vi "SCA-RT.vi"() -> ()   [LabVIEW 2016]
uses:
  controls/state control sample changer.ctl
  <vilib>/Platform/TimedLoop/XDataNode/timing_clust.ctl
  <vilib>/Platform/TimedLoop/XDataNode/nitl_modes.ctl
  <vilib>/Platform/TimedLoop/XDataNode/wakeup.ctl
  <vilib>/Analysis/baseanly.llb/Mean (DBL).vi
  <vilib>/Instr/_visa.llb/VISA Configure Serial Port (Instr).vi
  <vilib>/Motion/Express/_s/nimc.fb.read.readExecutionData.axis.vi
  <vilib>/Platform/TimedLoop/XDataNode/loadnilvce.vi
  <vilib>/Motion/Express/_s/nimc.fb.straightLineMove.startStraightLineMove.axis.modeAbsolute.0.vi
  <vilib>/Motion/Express/_s/nimc.fb.straightLineMove.startStraightLineMove.axis.modeRelative.0.vi
  <vilib>/Motion/BlockNode/FB.NIMotion.xnode
  <vilib>/Platform/TimedLoop/XDataNode/XDataNode.xnode
  <vilib>/Platform/TimedLoop/XDataNode/XDNodeRunTimeDep.lvlib
  <resource>/objmgr/nimcca.rc
  <vilib>/Analysis/NI_AALBase.lvlib
panel:
  out "Sample Rod DOWN":bool
  out "Sample Rod UP":bool
  out "SC GV CLOSED":bool
  out "SC GV OPEN":bool
  out "Retract Rod IN":bool
  out "Retract Rod OUT":bool
  out "Insert Rod IN":bool
  out "Insert Rod OUT":bool
  out "sample rod UP sensor":bool
  out "sample rod DOWN sensor":bool
  out "SC GV OPEN sensor":bool
  out "SC GV CLOSED sensor":bool
  out "insert rod IN sensor":bool
  out "insert rod OUT sensor":bool
  out "retract rod IN sensor":bool
  out "retract rod OUT sensor":bool
  out "Bellows IG 2":dbl
  out "Bellows CG 2":dbl
  out "Bellows CG 1":dbl
  out "Source CG 2":dbl
  out "Source CG 1":dbl
  out "Source IG1":dbl
  out "Bellows IG 1":dbl
  out "Source IG2":dbl
  out "CV 4":string
  out "CV 3":string
  out "ig 4":string
  out "ig 3":string
  out "CV 2":string
  out "CV 1":string
  out "ig 2":string
  out "cathode change":bool
  out "extractor current read":dbl
  out "extractor voltage read":dbl
  out "extractor set":dbl
  out "cathode voltage read":dbl
  out "cathode current":dbl
  out "cathode set":dbl
  in  "execute":bool
  out "Move (motor steps)":dbl
  out "Destination (encoder)":dbl
  in  "Window radius":u32=2
  out "In Range?":bool
  out "Lower Limit":u32
  out "Upper Limit":u32
  out "encoder position":u16
  out "change sample start end":bool
  out "start sample change":bool
  in  "clear error 3":bool
  in  "clear error 2":bool
  out "encoder set value":dbl
  out "done 2":bool
  out "set rod down 2":bool
  out "set cold cathode on 2":bool
  out "rotate wheel":bool
  out "set cold cathode on":bool
  out "set cold cathode off":bool
  out "set  vent source":bool
  out "set pump out system":bool
  out "set push out rod in":bool
  out "set push out rod out":bool
  out "set sc open":bool
  out "set sc close":bool
  out "set insert in":bool
  out "set insert out":bool
  out "set rod down":bool
  out "set rod up":bool
  out "Strings []":string[](array[string])
  out "wheel position readback":dbl
  out "position":dbl
  in  "clear error":bool
  out "action":string
  out "Axis Index":i32
  in  "end sample test":bool
  out "ig 1":string
  out "error out 8":errorcluster
  out "ig2":string
  out "error out 5":errorcluster
  out "convec":string
  out "Rod Up error out":errorcluster
  out "Retract Out 1 error out":errorcluster
  out "Retract In 1 error out":errorcluster
  out "indextest":dbl
  out "sc control":T1
  out "done":bool
  out "error out":errorcluster
  out "state control 2":T1
  in  "state control":T1="wait"
  in  "New Sample":dbl=1.0
  # "State Machine Sensors"
  # "Sensor Monitor Loop"
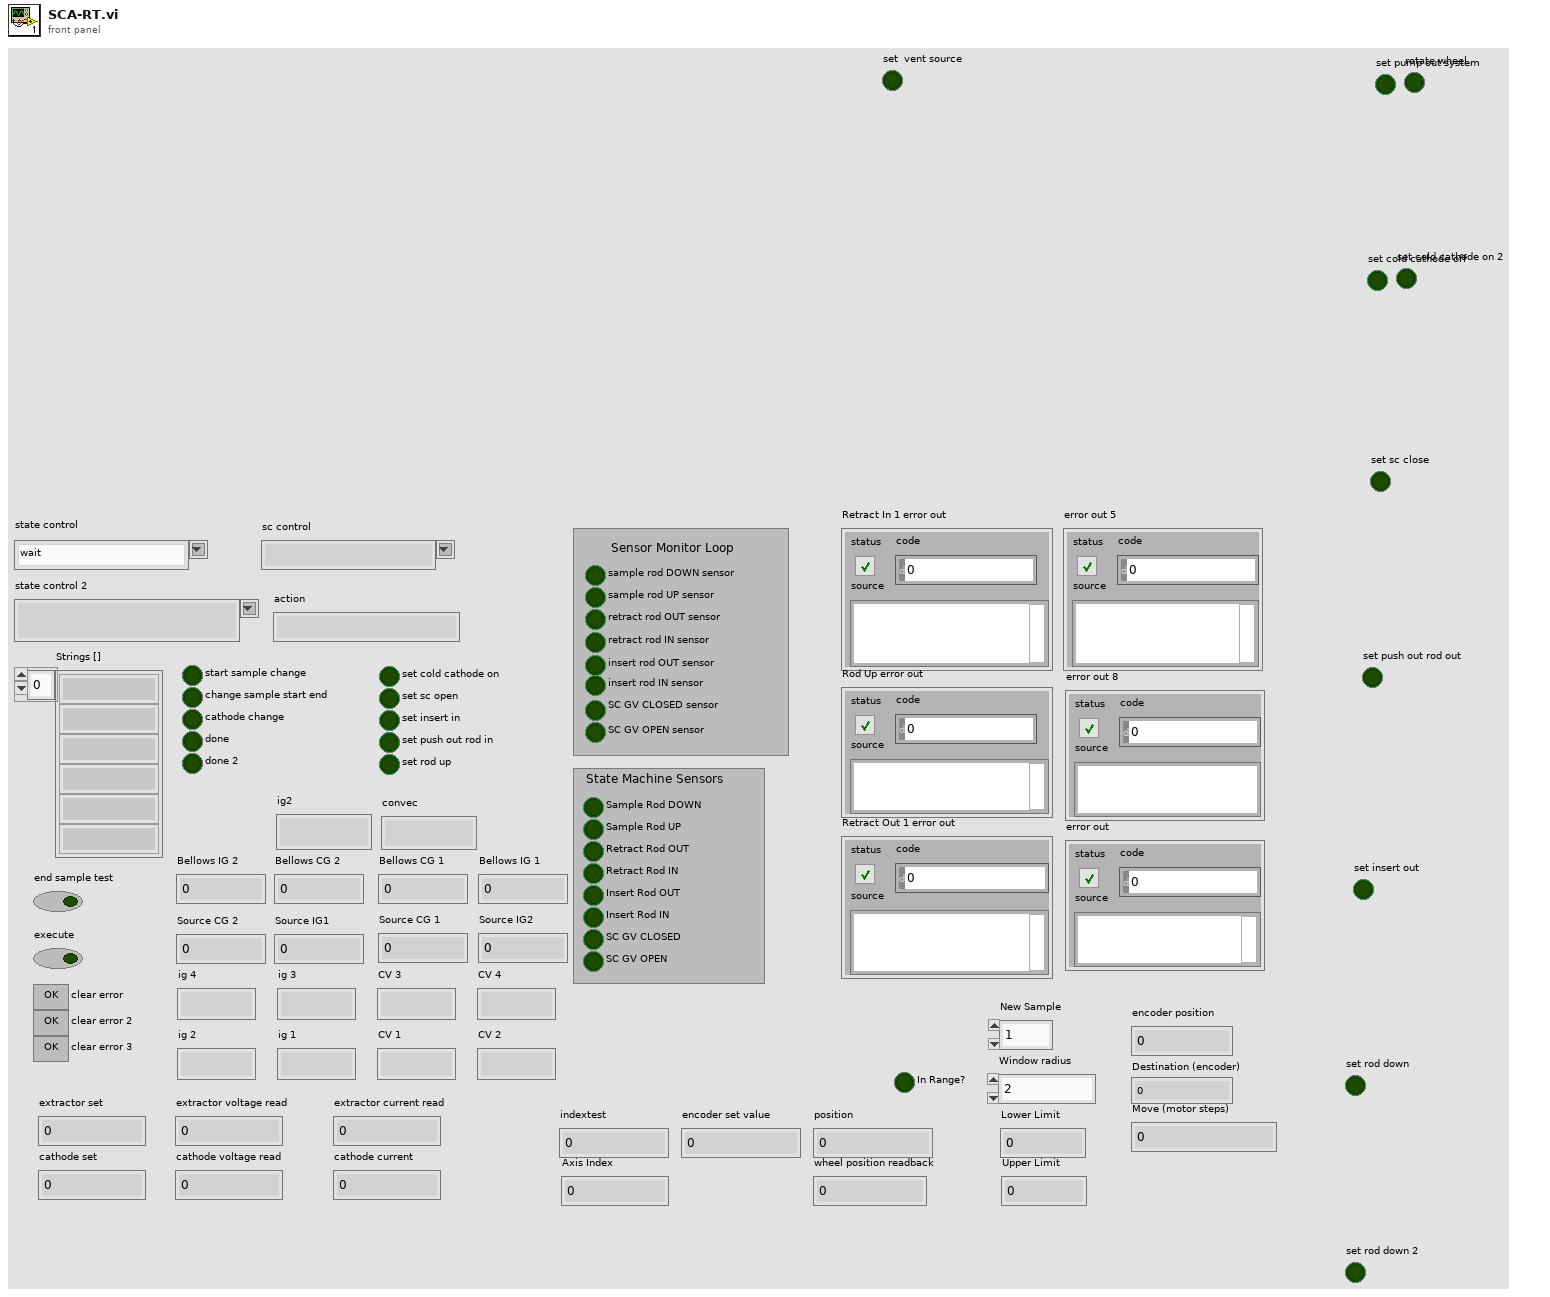
[diagram p1: front panel]
types:
  T1 = typedef "state control sample changer.ctl" = string
  T2 = typedef "XDNodeRunTimeDep.lvlib/timing_clust.ctl" = cluster{"Expected End [f-1]":u64, "Actual End [f-1]":u64, "Finished Late? [f-1]":bool, "Expected End [i-1]":u64, "Actual End [i-1]":u64, "Finished Late? [i-1]":bool, "Expected Start [i]":u64, "Actual Start [i]":u64, "Expected Start [f]":u64, "Actual Start [f]":u64, "Source Name":string, "Structure Name":string, "Period":i64, "Deadline":i64, "Offset":i64, "Start":i64, "Priority":i32, "Timeout":i32, "Mode":T3, "Wakeup Reason":T4, "Error":errorcluster, "Source Type":string, "Secondary Source Type":string, "Global End Time":u64, "Global Start Time":u64, "Frame Duration":u64, "Iteration Duration":u64, "Assigned CPU":i32, "I/O Scan Engine Mode":u32}
  T3 = typedef "XDNodeRunTimeDep.lvlib/nitl_modes.ctl" = enum32{"No Change", "Process missed periods, maintain original phase", "Discard missed periods, maintain original phase", "Process missed periods, ignore original phase", "Discard missed periods, ignore original phase"}
  T4 = typedef "XDNodeRunTimeDep.lvlib/wakeup.ctl" = enum32{"Normal", "Aborted", "Asynchronous wakeup", "Timing source error", "Timed loop error", "Timeout"}
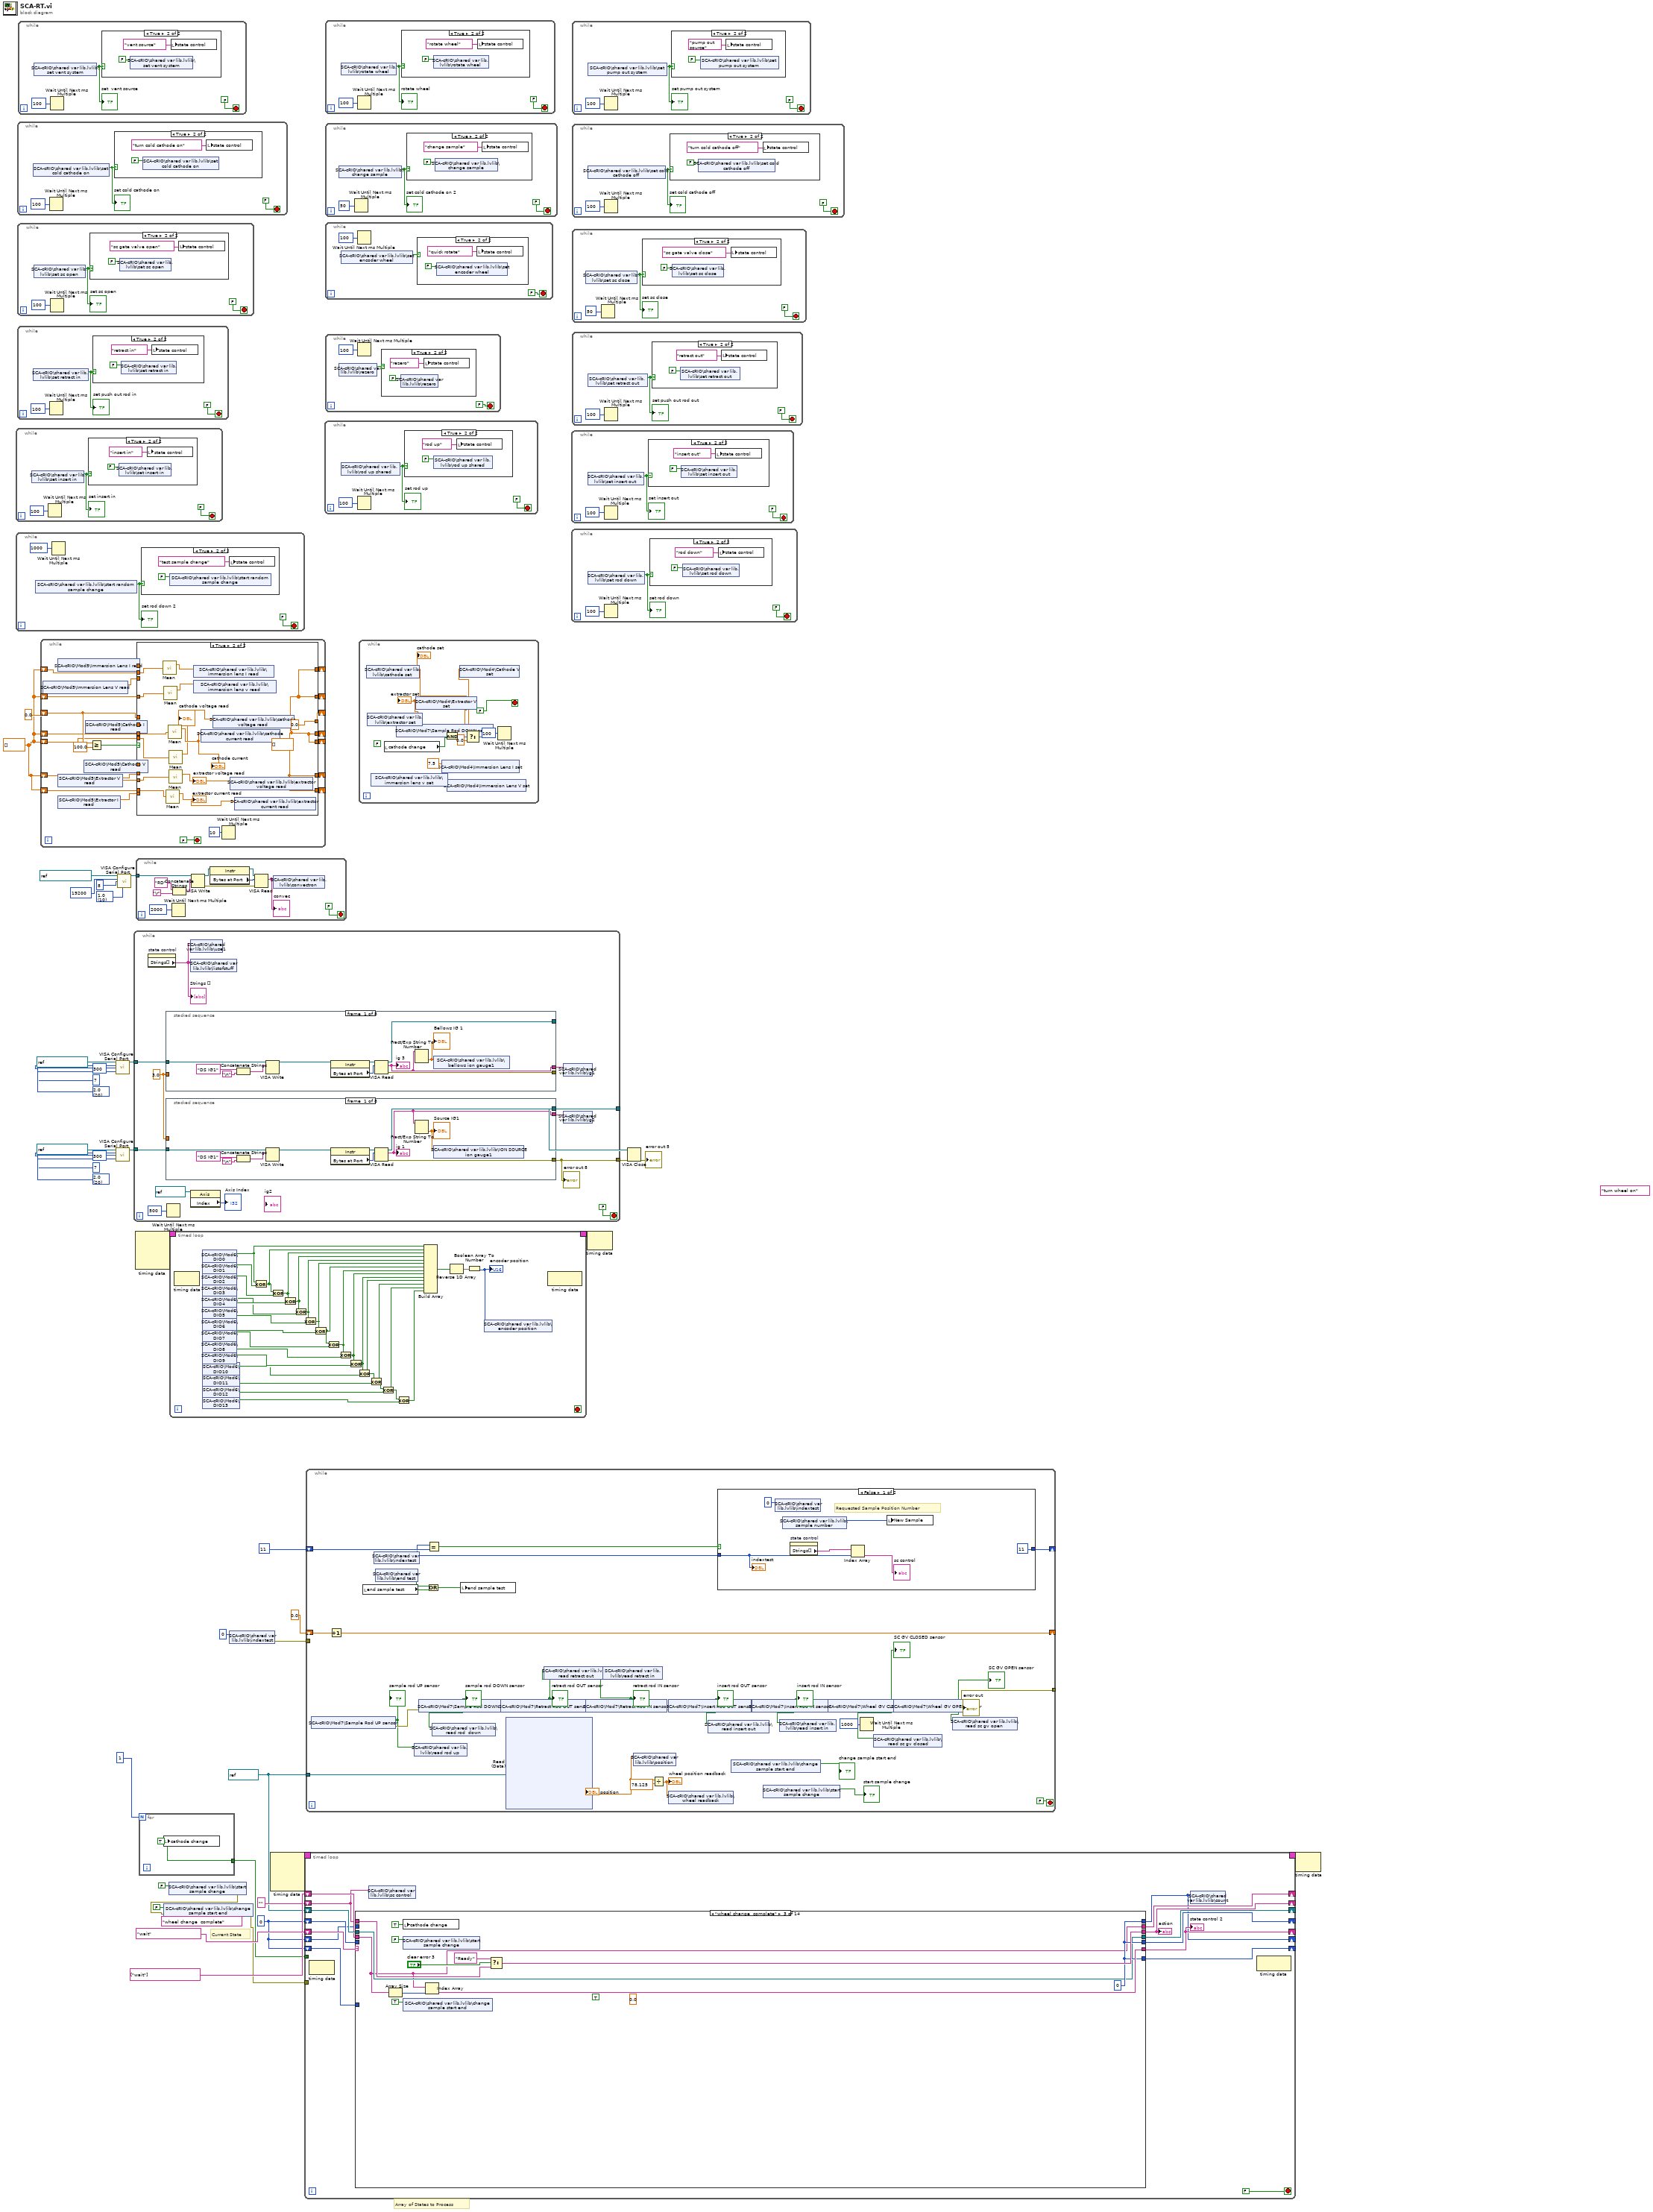
[diagram p0: block diagram]
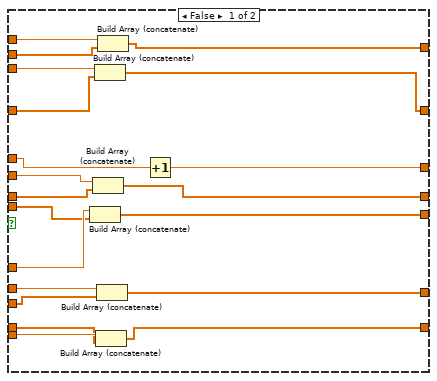
[diagram p2: hidden frame]
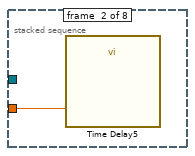
[diagram p20: hidden frame]
diagram:
  w1 = dbl[] []
  (unwired) T1 "wheel change  complete" ("state control")
  (unwired) T1 "turn wheel on" ("state control")
  w28 = u16 20 items=["1.0"=10, "1.5"=15, "2.0"=20] ("stop bits (10: 1 bit)")
  w32 = u16 10 items=["1.0"=10, "1.5"=15, "2.0"=20] ("stop bits (10: 1 bit)")
  w19 = u16 20 items=["1.0"=10, "1.5"=15, "2.0"=20] ("stop bits (10: 1 bit)")
  w13 = 0
  w12 = refnum<k21> "Axis 1" ("resource")
  # "Current State"
  # "Array of States to Process"
  n1 = while {
    stop <- FALSE stop-if-true
    n2 = shared-variable "SCA-cRIO\\shared var lib.lvlib\\set insert in"() -> (w41:bool)  [unwired: 1 in, 1 out]
    "set insert in" <- w41
    n3 = Wait Until Next ms Multiple(millisecond multiple=u32 100) -> ()  [unwired: 1 out]
    n4 = case shown="True" w41 {
      frame False {
      }
      frame True {
        n5 = shared-variable "SCA-cRIO\\shared var lib.lvlib\\set insert in"(FALSE ("rod up shared")) -> ()  [unwired: 1 in, 1 out]
        n6 = local write "state control"(T1 "insert in" ("state control")) -> ()
      }
    }
  }
  n7 = while {
    stop <- FALSE stop-if-true
    n8 = shared-variable "SCA-cRIO\\shared var lib.lvlib\\start random sample change"() -> (w46:bool)  [unwired: 1 in, 1 out]
    "set rod down 2" <- w46
    n9 = Wait Until Next ms Multiple(millisecond multiple=u32 1000) -> ()  [unwired: 1 out]
    n10 = case shown="True" w46 {
      frame False {
      }
      frame True {
        n11 = shared-variable "SCA-cRIO\\shared var lib.lvlib\\start random sample change"(FALSE ("rod up shared")) -> ()  [unwired: 1 in, 1 out]
        n12 = local write "state control"(T1 "test sample change" ("state control")) -> ()
      }
    }
  }
  n13 = while {
    stop <- FALSE stop-if-true
    n14 = shared-variable "SCA-cRIO\\shared var lib.lvlib\\set cold cathode on"() -> (w51:bool)  [unwired: 1 in, 1 out]
    "set cold cathode on" <- w51
    n15 = Wait Until Next ms Multiple(millisecond multiple=u32 100) -> ()  [unwired: 1 out]
    n16 = case shown="True" w51 {
      frame False {
      }
      frame True {
        n17 = shared-variable "SCA-cRIO\\shared var lib.lvlib\\set cold cathode on"(FALSE ("rod up shared")) -> ()  [unwired: 1 in, 1 out]
        n18 = local write "state control"(T1 "turn cold cathode on" ("state control")) -> ()
      }
    }
  }
  n19 = while {
    stop <- FALSE stop-if-true
    n20 = shared-variable "SCA-cRIO\\shared var lib.lvlib\\set retract in"() -> (w56:bool)  [unwired: 1 in, 1 out]
    "set push out rod in" <- w56
    n21 = Wait Until Next ms Multiple(millisecond multiple=u32 100) -> ()  [unwired: 1 out]
    n22 = case shown="True" w56 {
      frame False {
      }
      frame True {
        n23 = shared-variable "SCA-cRIO\\shared var lib.lvlib\\set retract in"(FALSE ("rod up shared")) -> ()  [unwired: 1 in, 1 out]
        n24 = local write "state control"(T1 "retract in" ("state control")) -> ()
      }
    }
  }
  n25 = while {
    stop <- FALSE stop-if-true
    n26 = shared-variable "SCA-cRIO\\shared var lib.lvlib\\set sc open"() -> (w61:bool)  [unwired: 1 in, 1 out]
    "set sc open" <- w61
    n27 = Wait Until Next ms Multiple(millisecond multiple=u32 100) -> ()  [unwired: 1 out]
    n28 = case shown="True" w61 {
      frame False {
      }
      frame True {
        n29 = shared-variable "SCA-cRIO\\shared var lib.lvlib\\set sc open"(FALSE ("rod up shared")) -> ()  [unwired: 1 in, 1 out]
        n30 = local write "state control"(T1 "sc gate valve open" ("state control")) -> ()
      }
    }
  }
  n31 = while {
    stop <- FALSE stop-if-true
    n32 = shared-variable "SCA-cRIO\\shared var lib.lvlib\\set vent system"() -> (w66:bool)  [unwired: 1 in, 1 out]
    "set  vent source" <- w66
    n33 = Wait Until Next ms Multiple(millisecond multiple=u32 100) -> ()  [unwired: 1 out]
    n34 = case shown="True" w66 {
      frame False {
      }
      frame True {
        n35 = shared-variable "SCA-cRIO\\shared var lib.lvlib\\set vent system"(FALSE ("rod up shared")) -> ()  [unwired: 1 in, 1 out]
        n36 = local write "state control"(T1 "vent source" ("state control")) -> ()
      }
    }
  }
  n37 = while {
    shift-right: [w86] -> _
    shift-left: 0.0 ("AI1") -> [w89]
    shift-right: [w84] -> _
    shift-left: w1 -> [w83]
    shift-right: [w85] -> _
    shift-left: w1 -> [w82]
    shift-right: [w80] -> _
    shift-left: w1 -> [w79]
    shift-right: [w77] -> _
    shift-left: w1 -> [w76]
    shift-right: [w71] -> _
    shift-left: w1 -> [w74]
    shift-right: [w70] -> _
    shift-left: w1 -> [w75]
    stop <- FALSE stop-if-true
    n38 = shared-variable "SCA-cRIO\\Mod5\\Immersion Lens V read"() -> (w72:dbl)  [unwired: 1 in, 1 out]
    n39 = shared-variable "SCA-cRIO\\Mod5\\Extractor V read"() -> (w81:dbl)  [unwired: 1 in, 1 out]
    n40 = shared-variable "SCA-cRIO\\Mod5\\Extractor I read"() -> (w78:dbl)  [unwired: 1 in, 1 out]
    n41 = shared-variable "SCA-cRIO\\Mod5\\Immersion Lens I read"() -> (w73:dbl)  [unwired: 1 in, 1 out]
    n42 = shared-variable "SCA-cRIO\\Mod5\\Cathode V read"() -> (w91:dbl)  [unwired: 1 in, 1 out]
    n43 = shared-variable "SCA-cRIO\\Mod5\\Cathode I read"() -> (w90:dbl)  [unwired: 1 in, 1 out]
    n44 = Greater Or Equal?(x=w89, y=100.0) -> (x >= y?=w87:bool)
    n45 = case shown="True" w87 {
      tunnel: w91 -> [w109 _]
      tunnel: w90 -> [w110 _]
      tunnel: w89 -> [w113 _]
      tunnel: [w112 0.0 ("AI1")] -> w86
      tunnel: [w111 w116] -> w85
      tunnel: [w108 w116] -> w84
      tunnel: w83 -> [w107 w125]
      tunnel: w82 -> [w106 w126]
      tunnel: w81 -> [w105 _]
      tunnel: [w104 w116] -> w80
      tunnel: w79 -> [w103 w124]
      tunnel: w78 -> [w102 _]
      tunnel: [w101 w116] -> w77
      tunnel: w76 -> [w100 w123]
      tunnel: w75 -> [w99 w115]
      tunnel: w74 -> [w98 w114]
      tunnel: w73 -> [w97 _]
      tunnel: w72 -> [w96 _]
      tunnel: [w95 w116] -> w71
      tunnel: [w94 w116] -> w70
      frame False {
        n46 = Build Array (concatenate)(w109, w107) -> (w108:dbl[])
        n47 = Build Array (concatenate)(w110, w106) -> (w111:dbl[])
        n48 = Build Array (concatenate)(w96, w99) -> (w94:dbl[])
        n49 = Build Array (concatenate)(w102, w100) -> (w101:dbl[])
        n50 = Build Array (concatenate)(w105, w103) -> (w104:dbl[])
        n51 = Build Array (concatenate)(w97, w98) -> (w95:dbl[])
        n52 = Increment(x=w113) -> (x+1=w112:dbl)
      }
      frame True {
        w116 = dbl[] []
        n53 = call-poly <vilib>:"Mean.vi"("X"=w114) -> ("mean"=w117:dbl)  [unwired: 1 out]
        n54 = call-poly <vilib>:"Mean.vi"("X"=w115) -> ("mean"=w118:dbl)  [unwired: 1 out]
        n55 = call-poly <vilib>:"Mean.vi"("X"=w123) -> ("mean"=w119:dbl)  [unwired: 1 out]
        "extractor current read" <- w119
        n56 = call-poly <vilib>:"Mean.vi"("X"=w126) -> ("mean"=w122:dbl)  [unwired: 1 out]
        "cathode current" <- w122
        n57 = call-poly <vilib>:"Mean.vi"("X"=w124) -> ("mean"=w120:dbl)  [unwired: 1 out]
        "extractor voltage read" <- w120
        n58 = call-poly <vilib>:"Mean.vi"("X"=w125) -> ("mean"=w121:dbl)  [unwired: 1 out]
        "cathode voltage read" <- w121
        n59 = shared-variable "SCA-cRIO\\shared var lib.lvlib\\immersion lens I read"(w117) -> ()  [unwired: 1 in, 1 out]
        n60 = shared-variable "SCA-cRIO\\shared var lib.lvlib\\immersion lens v read"(w118) -> ()  [unwired: 1 in, 1 out]
        n61 = shared-variable "SCA-cRIO\\shared var lib.lvlib\\cathode current read"(w122) -> ()  [unwired: 1 in, 1 out]
        n62 = shared-variable "SCA-cRIO\\shared var lib.lvlib\\cathode voltage read"(w121) -> ()  [unwired: 1 in, 1 out]
        n63 = shared-variable "SCA-cRIO\\shared var lib.lvlib\\extractor voltage read"(w120) -> ()  [unwired: 1 in, 1 out]
        n64 = shared-variable "SCA-cRIO\\shared var lib.lvlib\\extractor current read"(w119) -> ()  [unwired: 1 in, 1 out]
      }
    }
    n65 = Wait Until Next ms Multiple(millisecond multiple=u32 10) -> ()  [unwired: 1 out]
  }
  n66 = call-poly "VISA Configure Serial Port"("VISA resource name"=refnum<visa-resource-name> "ASRL8::INSTR", "baud rate (9600)"=u32 300, "data bits (8)"=u16 7, "stop bits (10: 1 bit)"=w28) -> ("VISA resource name out"=w29:refnum<visa-resource-name>)  [unwired: 10 in, 1 out]
  n67 = call-poly "VISA Configure Serial Port"("VISA resource name"=refnum<visa-resource-name> "ASRL6::INSTR", "baud rate (9600)"=u32 300, "data bits (8)"=u16 7, "stop bits (10: 1 bit)"=w19) -> ("VISA resource name out"=w20:refnum<visa-resource-name>)  [unwired: 10 in, 1 out]
  n68 = call-poly "VISA Configure Serial Port"("VISA resource name"=refnum<visa-resource-name> "ASRL7::INSTR", "baud rate (9600)"=u32 19200, "data bits (8)"=u16 8, "stop bits (10: 1 bit)"=w32) -> ("VISA resource name out"=w15:refnum<visa-resource-name>)  [unwired: 10 in, 1 out]
  n69 = while {
    tunnel: w20 -> [w138]
    tunnel: [w137] -> w21
    tunnel: [w136] -> w22
    tunnel: w29 -> [w130]
    stop <- FALSE ("stop 4") stop-if-true
    w129 = 3.0 ("Delay Time (s)")
    n70 = property on="state control" class="CmbBox (strict)"() -> ("Strings[]"=w132:string[])  [unwired: 2 in, 2 out]
    "Strings []" <- w132
    n71 = stacked-sequence {
      tunnel: w130 -> [w150 _ w160 _ w170 _ w180 _]
      tunnel: [w147 _ _ _ _ _ _ _] -> _
      tunnel: [w146 _ _ _ _ _ _ _] -> _
      tunnel: [w141 _ _ _ _ _ _ _] -> w128
      tunnel: w129 -> [_ w151 _ w161 _ w171 _ w181]
      frame #0 {
        n72 = Concatenate Strings("DS IG1" ("write buffer"), "\n") -> (w142:string)
        n73 = VISA Write(VISA resource name=w150, write buffer=w142) -> (VISA resource name out=w149:refnum<visa-resource-name>)  [unwired: 1 in, 2 out]
        n74 = property class="Instr"(reference=w149) -> (reference out=w148:refnum<visa-resource-name>, "Bytes at Port"=w144:u32)  [unwired: 1 in, 1 out]
        n75 = VISA Read(VISA resource name=w148, byte count=w144) -> (VISA resource name out=w147:refnum<visa-resource-name>, read buffer=w141:string, error out=w146:errorcluster)  [unwired: 1 in, 1 out]
        "ig 3" <- w141
        n76 = Fract/Exp String To Number(string=w141) -> (number=w140:dbl)  [unwired: 3 in, 1 out]
        "Bellows IG 1" <- w140
        n77 = shared-variable "SCA-cRIO\\shared var lib.lvlib\\bellows ion gauge1"(w140) -> ()  [unwired: 1 in, 1 out]
      }
      frame #1 {
        n78 = call "Time Delay5"("Delay Time (s)"=w151) -> ()  [unwired: 10 in, 1 out]
      }
      frame #2 {
        n79 = Concatenate Strings("DS IG2" ("write buffer"), "\n") -> (w154:string)
        n80 = VISA Write(VISA resource name=w160, write buffer=w154) -> (VISA resource name out=w159:refnum<visa-resource-name>)  [unwired: 1 in, 2 out]
        n81 = property class="Instr"(reference=w159) -> (reference out=w158:refnum<visa-resource-name>, "Bytes at Port"=w156:u32)  [unwired: 1 in, 1 out]
        n82 = VISA Read(VISA resource name=w158, byte count=w156) -> (read buffer=w153:string)  [unwired: 1 in, 3 out]
        "ig 4" <- w153
        n83 = Fract/Exp String To Number(string=w153) -> (number=w152:dbl)  [unwired: 3 in, 1 out]
        "Bellows IG 2" <- w152
        n84 = shared-variable "SCA-cRIO\\shared var lib.lvlib\\bellows ion gauge2"(w152) -> ()  [unwired: 1 in, 1 out]
      }
      frame #3 {
        n85 = call "Time Delay6"("Delay Time (s)"=w161) -> ()  [unwired: 10 in, 1 out]
      }
      frame #4 {
        n86 = Concatenate Strings("DS CG1" ("write buffer"), "\n") -> (w164:string)
        n87 = VISA Write(VISA resource name=w170, write buffer=w164) -> (VISA resource name out=w169:refnum<visa-resource-name>)  [unwired: 1 in, 2 out]
        n88 = property class="Instr"(reference=w169) -> (reference out=w168:refnum<visa-resource-name>, "Bytes at Port"=w166:u32)  [unwired: 1 in, 1 out]
        n89 = VISA Read(VISA resource name=w168, byte count=w166) -> (read buffer=w163:string)  [unwired: 1 in, 3 out]
        "CV 3" <- w163
        n90 = Fract/Exp String To Number(string=w163) -> (number=w162:dbl)  [unwired: 3 in, 1 out]
        "Bellows CG 1" <- w162
        n91 = shared-variable "SCA-cRIO\\shared var lib.lvlib\\Bellows covectron1"(w162) -> ()  [unwired: 1 in, 1 out]
      }
      frame #5 {
        n92 = call "Time Delay7"("Delay Time (s)"=w171) -> ()  [unwired: 10 in, 1 out]
      }
      frame #6 {
        n93 = Concatenate Strings("DS CG2" ("write buffer"), "\n") -> (w174:string)
        n94 = VISA Write(VISA resource name=w180, write buffer=w174) -> (VISA resource name out=w179:refnum<visa-resource-name>)  [unwired: 1 in, 2 out]
        n95 = property class="Instr"(reference=w179) -> (reference out=w178:refnum<visa-resource-name>, "Bytes at Port"=w176:u32)  [unwired: 1 in, 1 out]
        n96 = VISA Read(VISA resource name=w178, byte count=w176) -> (read buffer=w173:string)  [unwired: 1 in, 3 out]
        "CV 4" <- w173
        n97 = Fract/Exp String To Number(string=w173) -> (number=w172:dbl)  [unwired: 3 in, 1 out]
        "Bellows CG 2" <- w172
        n98 = shared-variable "SCA-cRIO\\shared var lib.lvlib\\Bellows covectron2"(w172) -> ()  [unwired: 1 in, 1 out]
      }
      frame #7 {
        n99 = call "Time Delay8"("Delay Time (s)"=w181) -> ()  [unwired: 10 in, 1 out]
      }
    }
    n100 = stacked-sequence {
      tunnel: w138 -> [w192 _ w202 _ w212 _ w222 _]
      tunnel: [w189 _ _ _ _ _ _ _] -> w137
      tunnel: [w188 _ _ _ _ _ _ _] -> w136
      tunnel: [w183 _ _ _ _ _ _ _] -> w131
      tunnel: w129 -> [_ w193 _ w203 _ w213 _ w223]
      frame #0 {
        n101 = Concatenate Strings("DS IG1" ("write buffer"), "\n") -> (w184:string)
        n102 = VISA Write(VISA resource name=w192, write buffer=w184) -> (VISA resource name out=w191:refnum<visa-resource-name>)  [unwired: 1 in, 2 out]
        n103 = property class="Instr"(reference=w191) -> (reference out=w190:refnum<visa-resource-name>, "Bytes at Port"=w186:u32)  [unwired: 1 in, 1 out]
        n104 = VISA Read(VISA resource name=w190, byte count=w186) -> (VISA resource name out=w189:refnum<visa-resource-name>, read buffer=w183:string, error out=w188:errorcluster)  [unwired: 1 in, 1 out]
        "ig 1" <- w183
        n105 = Fract/Exp String To Number(string=w183) -> (number=w182:dbl)  [unwired: 3 in, 1 out]
        "Source IG1" <- w182
        n106 = shared-variable "SCA-cRIO\\shared var lib.lvlib\\ION SOURCE ion gauge1"(w182) -> ()  [unwired: 1 in, 1 out]
      }
      frame #1 {
        n107 = call "Time Delay3"("Delay Time (s)"=w193) -> ()  [unwired: 10 in, 1 out]
      }
      frame #2 {
        n108 = Concatenate Strings("DS IG2" ("write buffer"), "\n") -> (w196:string)
        n109 = VISA Write(VISA resource name=w202, write buffer=w196) -> (VISA resource name out=w201:refnum<visa-resource-name>)  [unwired: 1 in, 2 out]
        n110 = property class="Instr"(reference=w201) -> (reference out=w200:refnum<visa-resource-name>, "Bytes at Port"=w198:u32)  [unwired: 1 in, 1 out]
        n111 = VISA Read(VISA resource name=w200, byte count=w198) -> (read buffer=w195:string)  [unwired: 1 in, 3 out]
        "ig 2" <- w195
        n112 = Fract/Exp String To Number(string=w195) -> (number=w194:dbl)  [unwired: 3 in, 1 out]
        "Source IG2" <- w194
        n113 = shared-variable "SCA-cRIO\\shared var lib.lvlib\\ION SOURCE ion gauge2"(w194) -> ()  [unwired: 1 in, 1 out]
      }
      frame #3 {
        n114 = call "Time Delay"("Delay Time (s)"=w203) -> ()  [unwired: 10 in, 1 out]
      }
      frame #4 {
        n115 = Concatenate Strings("DS CG1" ("write buffer"), "\n") -> (w206:string)
        n116 = VISA Write(VISA resource name=w212, write buffer=w206) -> (VISA resource name out=w211:refnum<visa-resource-name>)  [unwired: 1 in, 2 out]
        n117 = property class="Instr"(reference=w211) -> (reference out=w210:refnum<visa-resource-name>, "Bytes at Port"=w208:u32)  [unwired: 1 in, 1 out]
        n118 = VISA Read(VISA resource name=w210, byte count=w208) -> (read buffer=w205:string)  [unwired: 1 in, 3 out]
        "CV 1" <- w205
        n119 = Fract/Exp String To Number(string=w205) -> (number=w204:dbl)  [unwired: 3 in, 1 out]
        "Source CG 1" <- w204
        n120 = shared-variable "SCA-cRIO\\shared var lib.lvlib\\ION SOURCE covectron1"(w204) -> ()  [unwired: 1 in, 1 out]
      }
      frame #5 {
        n121 = call "Time Delay2"("Delay Time (s)"=w213) -> ()  [unwired: 10 in, 1 out]
      }
      frame #6 {
        n122 = Concatenate Strings("DS CG2" ("write buffer"), "\n") -> (w216:string)
        n123 = VISA Write(VISA resource name=w222, write buffer=w216) -> (VISA resource name out=w221:refnum<visa-resource-name>)  [unwired: 1 in, 2 out]
        n124 = property class="Instr"(reference=w221) -> (reference out=w220:refnum<visa-resource-name>, "Bytes at Port"=w218:u32)  [unwired: 1 in, 1 out]
        n125 = VISA Read(VISA resource name=w220, byte count=w218) -> (read buffer=w215:string)  [unwired: 1 in, 3 out]
        "CV 2" <- w215
        n126 = Fract/Exp String To Number(string=w215) -> (number=w214:dbl)  [unwired: 3 in, 1 out]
        "Source CG 2" <- w214
        n127 = shared-variable "SCA-cRIO\\shared var lib.lvlib\\ION SOURCE covectron2"(w214) -> ()  [unwired: 1 in, 1 out]
      }
      frame #7 {
        n128 = call "Time Delay4"("Delay Time (s)"=w223) -> ()  [unwired: 10 in, 1 out]
      }
    }
    "error out 8" <- w136
    n129 = Wait Until Next ms Multiple(millisecond multiple=u32 500) -> ()  [unwired: 1 out]
    n130 = shared-variable "SCA-cRIO\\shared var lib.lvlib\\use1"(w132) -> ()  [unwired: 1 in, 1 out]
    n131 = shared-variable "SCA-cRIO\\shared var lib.lvlib\\listofstuff"(w132) -> ()  [unwired: 1 in, 1 out]
    n132 = property class="Axis"(reference=refnum<k21> "Axis 1" ("resource")) -> ("Index"=→"Axis Index":i32)  [unwired: 1 in, 2 out]
    n133 = shared-variable "SCA-cRIO\\shared var lib.lvlib\\ig1"(w128) -> ()  [unwired: 1 in, 1 out]
    n134 = shared-variable "SCA-cRIO\\shared var lib.lvlib\\ig2"(w131) -> ()  [unwired: 1 in, 1 out]
  }
  n135 = node-c288() -> (w6:T2)  [unwired: 4 in]
  n136 = while {
    tunnel: w15 -> [w226]
    stop <- FALSE ("stop 3") stop-if-true
    n137 = Wait Until Next ms Multiple(millisecond multiple=u32 2000) -> ()  [unwired: 1 out]
    n138 = Concatenate Strings("RD" ("write buffer 2"), "\r") -> (w234:string)
    n139 = VISA Write(VISA resource name=w226, write buffer=w234) -> (VISA resource name out=w228:refnum<visa-resource-name>, error out=w227:errorcluster)  [unwired: 1 in, 1 out]
    n140 = property class="Instr"(reference=w228) -> (reference out=w229:refnum<visa-resource-name>, "Bytes at Port"=w230:u32)  [unwired: 1 in, 1 out]
    n141 = VISA Read(VISA resource name=w229, byte count=w230, error in (no error)=w227) -> (read buffer=w224:string)  [unwired: 3 out]
    "convec" <- w224
    n142 = shared-variable "SCA-cRIO\\shared var lib.lvlib\\convectron"(w224) -> ()  [unwired: 1 in, 1 out]
  }
  n143 = for {
    N: 1 -> [_]
    tunnel: [w235] -> w2
    w235 = TRUE ("cathode change")
    n144 = local write "cathode change"(w235) -> ()
  }
  n145 = shared-variable "SCA-cRIO\\shared var lib.lvlib\\start sample change"(FALSE ("start sample change")) -> (error out=w8:errorcluster)  [unwired: 1 in]
  n146 = shared-variable "SCA-cRIO\\shared var lib.lvlib\\change sample start end"(FALSE ("change sample start end"), error in=w8) -> (error out=w7:errorcluster)
  n147 = timed-loop {
    timing: w6 -> [_]
    timing-out: [_] -> w5
    stop <- _ stop-if-true
    n148 = node-c288() -> ()  [unwired: 1 in, 1 out]
    n149 = shared-variable "SCA-cRIO\\Mod6\\DIO0"() -> (w252:bool)  [unwired: 1 in, 1 out]
    n150 = shared-variable "SCA-cRIO\\Mod6\\DIO1"() -> (w251:bool)  [unwired: 1 in, 1 out]
    n151 = shared-variable "SCA-cRIO\\Mod6\\DIO2"() -> (w250:bool)  [unwired: 1 in, 1 out]
    n152 = shared-variable "SCA-cRIO\\Mod6\\DIO3"() -> (w249:bool)  [unwired: 1 in, 1 out]
    n153 = shared-variable "SCA-cRIO\\Mod6\\DIO4"() -> (w248:bool)  [unwired: 1 in, 1 out]
    n154 = shared-variable "SCA-cRIO\\Mod6\\DIO5"() -> (w247:bool)  [unwired: 1 in, 1 out]
    n155 = shared-variable "SCA-cRIO\\Mod6\\DIO6"() -> (w246:bool)  [unwired: 1 in, 1 out]
    n156 = shared-variable "SCA-cRIO\\Mod6\\DIO7"() -> (w245:bool)  [unwired: 1 in, 1 out]
    n157 = shared-variable "SCA-cRIO\\Mod6\\DIO8"() -> (w244:bool)  [unwired: 1 in, 1 out]
    n158 = shared-variable "SCA-cRIO\\Mod6\\DIO9"() -> (w243:bool)  [unwired: 1 in, 1 out]
    n159 = shared-variable "SCA-cRIO\\Mod6\\DIO10"() -> (w242:bool)  [unwired: 1 in, 1 out]
    n160 = shared-variable "SCA-cRIO\\Mod6\\DIO11"() -> (w241:bool)  [unwired: 1 in, 1 out]
    n161 = shared-variable "SCA-cRIO\\Mod6\\DIO12"() -> (w240:bool)  [unwired: 1 in, 1 out]
    n162 = shared-variable "SCA-cRIO\\Mod6\\DIO13"() -> (w239:bool)  [unwired: 1 in, 1 out]
    n163 = Exclusive Or(1:w251, 2:w252) -> (0:w253:bool)
    n164 = Exclusive Or(1:w250, 2:w253) -> (0:w254:bool)
    n165 = Exclusive Or(1:w249, 2:w254) -> (0:w255:bool)
    n166 = Exclusive Or(1:w248, 2:w255) -> (0:w256:bool)
    n167 = Exclusive Or(1:w247, 2:w256) -> (0:w257:bool)
    n168 = Exclusive Or(1:w246, 2:w257) -> (0:w258:bool)
    n169 = Exclusive Or(1:w245, 2:w258) -> (0:w259:bool)
    n170 = Exclusive Or(1:w244, 2:w259) -> (0:w260:bool)
    n171 = Exclusive Or(1:w243, 2:w260) -> (0:w261:bool)
    n172 = Exclusive Or(1:w242, 2:w261) -> (0:w262:bool)
    n173 = Exclusive Or(1:w241, 2:w262) -> (0:w263:bool)
    n174 = Exclusive Or(1:w240, 2:w263) -> (0:w264:bool)
    n175 = Exclusive Or(1:w239, 2:w264) -> (0:w265:bool)
    n176 = Build Array(w252, w253, w254, w255, w256, w257, w258, w259, w260, w261, w262, w263, w264, w265) -> (w237:bool[])
    n177 = Reverse 1D Array(array=w237) -> (reversed array=w236:bool[])
    n178 = Boolean Array To Number(Boolean array=w236) -> (number=w238:u32)
    "encoder position" <- w238
    n179 = shared-variable "SCA-cRIO\\shared var lib.lvlib\\encoder position"(w238) -> ()  [unwired: 1 in, 1 out]
    n180 = node-c288() -> ()  [unwired: 1 in, 1 out]
  }
  n181 = shared-variable "SCA-cRIO\\shared var lib.lvlib\\indextest"(i16 0 ("indextest")) -> (error out=w33:errorcluster)  [unwired: 1 in]
  n182 = node-c288() -> (w39:T2)  [unwired: 4 in]
  n183 = timed-loop {
    timing: w39 -> [_]
    timing-out: [_] -> w38
    shift-right: [w280] -> _
    shift-left: w12 -> [w281]
    shift-right: [w278] -> _
    shift-left: T1 "wait" ("state control") -> [w279]
    shift-right: [w274] -> _
    shift-left: T1[] ["wait"] -> [w277]
    shift-right: [w275] -> _
    shift-left: w13 -> [w276]
    shift-right: [w273] -> _
    shift-left: "" -> [w270]
    shift-right: [w271] -> _
    shift-left: w13 -> [w272]
    shift-right: [w268] -> _
    shift-left: w13 -> [w269]
    tunnel: w7 -> [_]
    tunnel: w2 -> [_]
    stop <- FALSE ("stop 2") stop-if-true
    n184 = node-c288() -> ()  [unwired: 1 in, 1 out]
    n185 = case shown="\"wheel change  complete\"" w279 {
      selector: w279 -> [_ _ _ w378 w420 w449 w487 w523 _ _ w613 w677 w743 w767]
      tunnel: w281 -> [w293 w353 w365 w400 w438 w476 w512 w542 w558 w609 w640 w681 w728 w788]
      tunnel: [w293 w353 w365 w400 w438 w476 w512 w542 w557 w609 w639 w681 w728 w787] -> w280
      tunnel: [w283 w359 w371 w381 w422 w453 w492 w529 w556 w599 w629 w679 w744 w768] -> w278
      tunnel: w277 -> [w292 w351 w362 w379 w421 w448 w488 w522 w555 w611 w614 w676 w704 w771]
      tunnel: w276 -> [_ _ _ w388 w432 w463 w500 _ _ w605 w636 w693 w726 w783]
      tunnel: [w286 w354 w366 w387 w428 w460 w499 w532 w553 w604 w637 w694 w726 w784] -> w275
      tunnel: [w284 w351 w362 w382 w412 w456 w491 w530 w555 w611 w630 w690 w746 w770] -> w274
      tunnel: w270 -> [w289 w357 w369 _ _ _ _ _ _ _ _ _ _ _]
      tunnel: [w288 w356 w368 w377 w424 w455 w490 w538 "wheel off" ("y") "sample changer test" ("y") w628 w689 w742 w766] -> w273
      tunnel: w272 -> [_ _ _ w383 w419 w452 w495 w536 _ _ w631 w691 _ w772]
      tunnel: [w286 w354 w366 w376 w415 w451 w494 w527 w553 0 w622 w684 0 ("t") w760] -> w271
      tunnel: w269 -> [_ _ _ w375 w414 w450 w489 w526 w552 w592 w627 w688 w741 w765]
      tunnel: [w286 w354 w366 w375 w414 w450 w489 w526 w552 w591 w627 w688 w741 w765] -> w268
      frame "wait", Default {
        w286 = 0
        n186 = Select(t="Ready", s="clear error", f=w289) -> (s? t:f=w288:string)
        n187 = case shown="\"rod up\"" "state control" {
          tunnel: w292 -> [_ _ _ _ _ _ _ _ _ _ _ _ _ _ _ _ _ _]
          tunnel: [w294 w297 w300 w303 w306 w309 w312 w315 w318 w321 w325 w328 w331 w334 w337 w339 w342 w347] -> w284
          tunnel: "state control" -> [_ _ _ _ _ _ _ _ _ _ _ _ _ _ _ _ _ _]
          tunnel: [w295 w298 w301 w304 w307 w310 w313 w316 w319 w322 w324 w327 w330 w333 w336 w340 w343 w345] -> _
          frame "sc gate valve close" {
            w294 = T1[] ["sc gate valve close"]
            n188 = Index Array(array=w294, index=0) -> (element=w295:T1)
          }
          frame "sc gate valve open" {
            w297 = T1[] ["sc gate valve open"]
            n189 = Index Array(array=w297, index=0) -> (element=w298:T1)
          }
          frame "rod up" {
            w300 = T1[] ["rod up"]
            n190 = Index Array(array=w300, index=0) -> (element=w301:T1)
          }
          frame "rod down" {
            w303 = T1[] ["rod down"]
            n191 = Index Array(array=w303, index=0) -> (element=w304:T1)
          }
          frame "retract in" {
            w306 = T1[] ["retract in"]
            n192 = Index Array(array=w306, index=0) -> (element=w307:T1)
          }
          frame "retract out" {
            w309 = T1[] ["retract out"]
            n193 = Index Array(array=w309, index=0) -> (element=w310:T1)
          }
          frame "insert in" {
            w312 = T1[] ["insert in"]
            n194 = Index Array(array=w312, index=0) -> (element=w313:T1)
          }
          frame "insert out" {
            w315 = T1[] ["insert out"]
            n195 = Index Array(array=w315, index=0) -> (element=w316:T1)
          }
          frame "turn cold cathode on" {
            w318 = T1[] ["turn cold cathode on"]
            n196 = Index Array(array=w318, index=0) -> (element=w319:T1)
          }
          frame "turn cold cathode off" {
            w321 = T1[] ["turn cold cathode off"]
            n197 = Index Array(array=w321, index=0) -> (element=w322:T1)
          }
          frame "rotate wheel" {
            w325 = T1[] ["check position"]
            n198 = Index Array(array=w325, index=0) -> (element=w324:T1)
          }
          frame "change sample" {
            w328 = T1[] ["wheel change start", "rod up", "retract in", "retract out", "check position", "insert in", "insert out", "rod down", "wheel change  complete"]
            n199 = Index Array(array=w328, index=0) -> (element=w327:T1)
          }
          frame "test sample change" {
            w331 = T1[] ["rod up", "retract in", "retract out", "check position", "insert in", "insert out", "rod down", "test sample change"]
            n200 = Index Array(array=w331, index=0) -> (element=w330:T1)
          }
          frame "vent source" {
            w334 = T1[] ["turn cold cathode off", "rod up", "retract in", "retract out", "insert out", "sc gate valve close"]
            n201 = Index Array(array=w334, index=0) -> (element=w333:T1)
          }
          frame "pump out source" {
            w337 = T1[] ["sc gate valve open", "rod up", "check position", "insert in", "insert out", "rod down"]
            n202 = Index Array(array=w337, index=0) -> (element=w336:T1)
          }
          frame "wait", Default {
            w339 = T1[] ["wait"]
            n203 = Index Array(array=w339, index=0) -> (element=w340:T1)
          }
          frame "quick rotate" {
            w342 = T1[] ["quick rotate"]
            n204 = Index Array(array=w342, index=0) -> (element=w343:T1)
          }
          frame "rezero" {
            w347 = T1[] ["rezero"]
            n205 = Index Array(array=w347, index=0) -> (element=w345:T1)
          }
        }
        n206 = Index Array(array=w284, index=0) -> (element=w283:T1)
      }
      frame "wheel change start" {
        (unwired) 0.0 ("position")
        w354 = 0
        n207 = shared-variable "SCA-cRIO\\shared var lib.lvlib\\start sample change"(TRUE ("start sample change")) -> ()  [unwired: 1 in, 1 out]
        n208 = shared-variable "SCA-cRIO\\shared var lib.lvlib\\change sample start end"(FALSE ("change sample start end")) -> ()  [unwired: 1 in, 1 out]
        n209 = Select(t="Ready", s="clear error 2", f=w357) -> (s? t:f=w356:string)
        n210 = Index Array(array=w351, index=1) -> (element=w359:T1)
        "cathode change" <- FALSE ("execute")
      }
      frame "wheel change  complete" {
        (unwired) 0.0 ("position")
        (unwired) TRUE ("execute")
        w366 = 0
        n211 = Array Size(array=w362) -> (size(s)=w361:i32)
        n212 = local write "cathode change"(TRUE ("execute")) -> ()
        n213 = shared-variable "SCA-cRIO\\shared var lib.lvlib\\start sample change"(FALSE ("start sample change")) -> ()  [unwired: 1 in, 1 out]
        n214 = shared-variable "SCA-cRIO\\shared var lib.lvlib\\change sample start end"(TRUE ("change sample start end")) -> ()  [unwired: 1 in, 1 out]
        n215 = Index Array(array=w362, index=w361) -> (element=w371:T1)
        n216 = Select(t="Ready", s="clear error 3", f=w369) -> (s? t:f=w368:string)
      }
      frame "sc gate valve close", "sc gate valve open" {
        (unwired) T1 "wait" ("state control")
        n217 = Search 1D Array(1D array=w379, element=w378) -> (index of element=w395:i32)  [unwired: 1 in]
        n218 = Increment(x=w395) -> (x+1=w394:i32)
        n219 = Index Array(array=w379, index=w394) -> (element=w396:T1)
        n220 = local write "state control"(w396) -> ()
        n221 = shared-variable "SCA-cRIO\\Mod7\\Wheel GV OPEN sensor"() -> (w385:bool)  [unwired: 1 in, 1 out]
        "SC GV OPEN" <- w385
        n222 = shared-variable "SCA-cRIO\\Mod7\\Wheel GV CLOSED sensor"() -> (w386:bool)  [unwired: 1 in, 1 out]
        "SC GV CLOSED" <- w386
        n223 = Equal?(x=w378, y="sc gate valve close") -> (x = y?=w374:bool)
        n224 = case shown="True" w374 {
          frame False {
          }
          frame True {
            n225 = shared-variable "SCA-cRIO\\Mod8\\Extractor HV Enable"(FALSE ("cold cathode")) -> ()  [unwired: 1 in, 1 out]
          }
        }
        n226 = Select(t=FALSE ("sc gate valve"), s=w374, f=TRUE ("sc gate valve")) -> (s? t:f=w372:bool)
        n227 = shared-variable "SCA-cRIO\\Mod8\\Wheel GV Actuator"(w372) -> ()  [unwired: 1 in, 1 out]
        n228 = Select(t=w385, s=w372, f=w386) -> (s? t:f=w390:bool)
        n229 = Select(t=w388, s=w390, f=0) -> (s? t:f=w392:i32)
        n230 = Increment(x=w392) -> (x+1=w387:i32)
        n231 = Greater Or Equal?(x=w387, y=70) -> (x >= y?=w389:bool)
        n232 = Select(t=w396, s=w389, f=w378) -> (s? t:f=w380:T1)
        n233 = Increment(x=w383) -> (x+1=w376:i32)
        n234 = Greater Or Equal?(x=w376, y=200) -> ()  [unwired: 1 out]
        n235 = case shown="True" FALSE {
          tunnel: [w403 0] -> _
          tunnel: [w404 T1[] ["wait", "insert out", "rod up", "wait"]] -> w382
          tunnel: [w405 T1 "wait" ("state control")] -> w381
          tunnel: w380 -> [w405 _]
          tunnel: w379 -> [w404 _]
          tunnel: w376 -> [w403 _]
          tunnel: w378 -> [w402 _]
          tunnel: [w402 "gate valve failure"] -> w377
          frame False {
          }
          frame True {
          }
        }
      }
      frame "rod down", "rod up" {
        n236 = call "Extract-State-from-Array-of-States.vi"("Current State"=w420, "Array of States to Process"=w421) -> ("Modified Array of States to Process"=w434:T1)  [unwired: 13 in]
        n237 = shared-variable "SCA-cRIO\\Mod7\\Sample Rod UP sensor"() -> (w425:bool, error out=→"Rod Up error out":errorcluster)  [unwired: 1 in]
        "Sample Rod UP" <- w425
        n238 = Equal?(x=w420, y="rod down") -> (x = y?=w436:bool)
        n239 = shared-variable "SCA-cRIO\\Mod7\\Sample Rod DOWN sensor"() -> (w413:bool)  [unwired: 1 in, 1 out]
        "Sample Rod DOWN" <- w413
        n240 = Select(t=TRUE ("sc gate valve"), s=w436, f=FALSE ("sc gate valve")) -> (s? t:f=w411:bool)
        n241 = shared-variable "SCA-cRIO\\shared var lib.lvlib\\sample change complete"(w413) -> ()  [unwired: 1 in, 1 out]
        n242 = shared-variable "SCA-cRIO\\Mod8\\Sample Rod Actuator"(w411) -> ()  [unwired: 1 in, 1 out]
        n243 = shared-variable "SCA-cRIO\\Mod8\\Extractor HV Enable"(w411) -> ()  [unwired: 1 in, 1 out]
        n244 = Select(t=w413, s=w411, f=w425) -> (s? t:f=w433:bool)
        n245 = Select(t=w432, s=w433, f=0) -> (s? t:f=w429:i32)
        n246 = local write "state control"(w434) -> ()
        n247 = Increment(x=w419) -> (x+1=w416:i32)
        n248 = Increment(x=w429) -> (x+1=w428:i32)
        n249 = Greater Or Equal?(x=w428, y=10) -> (x >= y?=w430:bool)
        n250 = Select(t=w434, s=w430, f=w420) -> (s? t:f=w423:T1)
        n251 = Greater Or Equal?(x=w416, y=1000) -> (x >= y?=w417:bool)
        n252 = case shown="False" w417 {
          tunnel: [w442 0] -> w415
          tunnel: [w439 T1[] ["wait", "insert out", "wait"]] -> w412
          tunnel: [w440 T1 "wait" ("state control")] -> w422
          tunnel: w416 -> [w442 _]
          tunnel: w420 -> [w441 _]
          tunnel: [w441 "rod failure"] -> w424
          tunnel: w423 -> [w440 _]
          tunnel: w421 -> [w439 _]
          frame False {
          }
          frame True {
          }
        }
      }
      frame "retract in", "retract out" {
        n253 = call "Extract-State-from-Array-of-States.vi"("Current State"=w449, "Array of States to Process"=w448) -> ("Modified Array of States to Process"=w447:T1)  [unwired: 13 in]
        n254 = Equal?(x=w449, y="retract in") -> (x = y?=w474:bool)
        n255 = shared-variable "SCA-cRIO\\Mod7\\Retract Rod OUT sensor"() -> (w469:bool, error out=→"Retract Out 1 error out":errorcluster)  [unwired: 1 in]
        "Retract Rod OUT" <- w469
        n256 = shared-variable "SCA-cRIO\\Mod7\\Retract Rod IN sensor"() -> (w470:bool, error out=→"Retract In 1 error out":errorcluster)  [unwired: 1 in]
        "Retract Rod IN" <- w470
        n257 = Select(t=TRUE ("sc gate valve"), s=w474, f=FALSE ("sc gate valve")) -> (s? t:f=w471:bool)
        n258 = shared-variable "SCA-cRIO\\Mod8\\Retract Rod Actuator"(w471) -> ()  [unwired: 1 in, 1 out]
        n259 = Select(t=w470, s=w471, f=w469) -> (s? t:f=w462:bool)
        n260 = Select(t=w463, s=w462, f=0) -> (s? t:f=w465:i32)
        n261 = local write "state control"(w447) -> ()
        n262 = Increment(x=w465) -> (x+1=w460:i32)
        n263 = Increment(x=w452) -> (x+1=w457:i32)
        n264 = Greater Or Equal?(x=w460, y=30) -> (x >= y?=w461:bool)
        n265 = Greater Or Equal?(x=w457, y=200) -> (x >= y?=w458:bool)
        n266 = Select(t=w447, s=w461, f=w449) -> (s? t:f=w454:T1)
        n267 = case shown="False" w458 {
          tunnel: [w480 0] -> w451
          tunnel: [w477 T1[] ["retract out", "insert out", "wait"]] -> w456
          tunnel: [w478 T1 "retract out" ("state control")] -> w453
          tunnel: w457 -> [w480 _]
          tunnel: w449 -> [w479 _]
          tunnel: [w479 "retract failure"] -> w455
          tunnel: w454 -> [w478 _]
          tunnel: w448 -> [w477 _]
          frame False {
          }
          frame True {
          }
        }
      }
      frame "insert in", "insert out" {
        n268 = call "Extract-State-from-Array-of-States.vi"("Current State"=w487, "Array of States to Process"=w488) -> ("Modified Array of States to Process"=w485:T1)  [unwired: 13 in]
        n269 = Equal?(x=w487, y="insert in") -> (x = y?=w510:bool)
        n270 = shared-variable "SCA-cRIO\\Mod7\\Insert Rod OUT sensor"() -> (w505:bool)  [unwired: 1 in, 1 out]
        "Insert Rod OUT" <- w505
        n271 = shared-variable "SCA-cRIO\\Mod7\\Insert Rod IN sensor"() -> (w506:bool)  [unwired: 1 in, 1 out]
        "Insert Rod IN" <- w506
        n272 = Select(t=TRUE ("sc gate valve"), s=w510, f=FALSE ("sc gate valve")) -> (s? t:f=w507:bool)
        n273 = shared-variable "SCA-cRIO\\Mod8\\Insert Rod Actuator"(w507) -> ()  [unwired: 1 in, 1 out]
        n274 = Select(t=w506, s=w507, f=w505) -> (s? t:f=w501:bool)
        n275 = Select(t=w500, s=w501, f=0) -> (s? t:f=w503:i32)
        n276 = local write "state control"(w485) -> ()
        n277 = Increment(x=w503) -> (x+1=w499:i32)
        n278 = Increment(x=w495) -> (x+1=w496:i32)
        n279 = Greater Or Equal?(x=w499, y=30) -> (x >= y?=w486:bool)
        n280 = Greater Or Equal?(x=w496, y=500) -> (x >= y?=w497:bool)
        n281 = Select(t=w485, s=w486, f=w487) -> (s? t:f=w493:T1)
        n282 = case shown="False" w497 {
          tunnel: [w516 0] -> w494
          tunnel: [w513 T1[] ["retract out", "insert out", "wait"]] -> w491
          tunnel: [w514 T1 "insert out" ("state control")] -> w492
          tunnel: w496 -> [w516 _]
          tunnel: w487 -> [w515 _]
          tunnel: [w515 "insert failure"] -> w490
          tunnel: w493 -> [w514 _]
          tunnel: w488 -> [w513 _]
          frame False {
          }
          frame True {
          }
        }
      }
      frame "turn cold cathode off", "turn cold cathode on" {
        w524 = TRUE ("sc gate valve")
        n283 = disable-structure shown="Disabled" {
          frame Disabled {
            # "Unused Code (Kubley)"
            n284 = local read "ig2"() -> (w543:string)
            n285 = Fract/Exp String To Number(string=w543) -> (number=w544:dbl)  [unwired: 3 in, 1 out]
            n286 = Less Or Equal?(x=w544, y=0.001) -> ()  [unwired: 1 out]
          }
          frame Enabled {
          }
        }
        n287 = call "Extract-State-from-Array-of-States.vi"("Current State"=w523, "Array of States to Process"=w522) -> ("Modified Array of States to Process"=w521:T1)  [unwired: 13 in]
        n288 = Equal?(x=w523, y="turn cold cathode on") -> (x = y?=w534:bool)
        n289 = local write "state control"(w521) -> ()
        n290 = Select(t=w521, s=w524, f=T1 "turn cold cathode on" ("state control")) -> (s? t:f=w533:T1)
        n291 = Select(t=w524, s=w534, f=FALSE ("sc gate valve")) -> (s? t:f=w525:bool)
        n292 = shared-variable "SCA-cRIO\\Mod8\\Extractor HV Enable"(w525) -> ()  [unwired: 1 in, 1 out]
        n293 = Select(t=w523, s=w524, f="PRESSURE TO HIGH, COLD CATHODE OFF" ("y")) -> (s? t:f=w538:string)
        n294 = Select(t=w533, s=w534, f=w533) -> (s? t:f=w528:T1)
        n295 = Increment(x=w536) -> (x+1=w527:i32)
        n296 = Greater Or Equal?(x=w527, y=500) -> (x >= y?=w531:bool)
        n297 = case shown="False" w531 {
          tunnel: [w547 0] -> w532
          tunnel: [w548 T1[] ["wait", "insert out", "rod up", "wait"]] -> w530
          tunnel: w522 -> [w548 _]
          tunnel: w527 -> [w547 _]
          tunnel: [w546 T1 "wait" ("state control")] -> w529
          tunnel: w528 -> [w546 _]
          frame False {
          }
          frame True {
          }
        }
      }
      frame "turn wheel off", "turn wheel on" {
        w553 = 0
        w556 = T1 "wait" ("state control")
        (unwired) TRUE ("execute")
        n298 = xnode "Straight-Line Move"("resource"=w558, "execute"=FALSE) -> ("resource out"=w557:refnum<k21>)  [unwired: 8 in, 5 out]
        n299 = local write "state control"(w556) -> ()
      }
      frame "test sample change" {
        n300 = Random Number (0-1)() -> (number: 0 to 1=w598:dbl)
        n301 = Multiply(x=w598, y=63.0) -> (x*y=w596:dbl)
        n302 = Greater Or Equal?(x=w605, y=150) -> (x >= y?=w606:bool)
        n303 = Round Toward +Infinity(x=w596) -> (ceil(x): smallest int >= x=w595:dbl)
        n304 = shared-variable "SCA-cRIO\\shared var lib.lvlib\\sample number"(w595) -> ()  [unwired: 1 in, 1 out]
        n305 = Increment(x=w605) -> (x+1=w604:i32)
        n306 = Increment(x=w592) -> (x+1=w591:i32)
        n307 = shared-variable "SCA-cRIO\\shared var lib.lvlib\\stop random sample change"() -> (w587:bool)  [unwired: 1 in, 1 out]
        n308 = Index Array(array=T1[] ["rod up", "retract in", "retract out", "rotate wheel", "insert in", "insert out", "rod down", "rod up"], index=0) -> (element=w603:T1)
        n309 = Select(t=w603, s=w606, f=T1 "test sample change" ("state control")) -> (s? t:f=w601:T1)
        n310 = Or(x="end sample test", y=w587) -> (x .or. y?=w586:bool)
        n311 = Select(t=T1 "wait", s=w586, f=w601) -> (s? t:f=w599:T1)
        n312 = And(x=w586, y=FALSE) -> (x .and. y?=w588:bool)
        n313 = local write "state control"(w599) -> ()
        n314 = shared-variable "SCA-cRIO\\shared var lib.lvlib\\stop random sample change"(w588) -> ()  [unwired: 1 in, 1 out]
      }
      frame "rotate wheel" {
        w635 = 350 ("y")
        w638 = 10000.0 ("acceleration")
        # "Motor Value"
        n315 = call "Extract-State-from-Array-of-States.vi"("Current State"=w613, "Array of States to Process"=w614) -> ("Modified Array of States to Process"=w612:T1)  [unwired: 13 in]
        n316 = Increment(x=w636) -> (x+1=w637:i32)
        n317 = Greater Or Equal?(x=w637, y=w635) -> (x >= y?=w625:bool)
        n318 = Subtract(x=w635, y=5) -> (x-y=w626:i32)
        n319 = Less Or Equal?(x=w636, y=w626) -> ()  [unwired: 1 out]
        n320 = local write "state control"(w612) -> ()
        n321 = local read "Move (motor steps)"() -> (w618:dbl)
        n322 = shared-variable "SCA-cRIO\\shared var lib.lvlib\\motor value"(w618) -> ()  [unwired: 1 in, 1 out]
        n323 = xnode "Straight-Line Move"("resource"=w640, "execute"="execute", "position"=w618, "velocity"=w638, "acceleration"=w638, "deceleration"=w638, "accel. jerk"=w638, "smoothing"=w638) -> ("resource out"=w639:refnum<k21>, "done"=w615:bool)  [unwired: 2 in, 4 out]
        "done" <- w615
        n324 = Increment(x=w631) -> (x+1=w624:i32)
        n325 = Select(t=0, s=w625, f=w624) -> (s? t:f=w622:i32)
        n326 = Greater Or Equal?(x=w624, y=800) -> (x >= y?=w632:bool)
        n327 = Select(t=T1 "wait position" ("f"), s=w615, f=T1 "rotate wheel") -> (s? t:f=w619:T1)
        n328 = Not(x=w615) -> (.not. x?=w616:bool)
        n329 = case shown="False" w632 {
          tunnel: [w644 0] -> _
          tunnel: [w641 T1[] ["retract out", "insert out", "wait"]] -> w630
          tunnel: [w642 T1 "retract out" ("state control")] -> w629
          tunnel: w624 -> [w644 _]
          tunnel: w613 -> [w643 _]
          tunnel: [w643 "rotate failure"] -> w628
          tunnel: w619 -> [w642 _]
          tunnel: w614 -> [w641 _]
          frame False {
          }
          frame True {
          }
        }
        n330 = local write "execute"(w616) -> ()
      }
      frame "wait position" {
        n331 = call "Extract-State-from-Array-of-States.vi"("Current State"=w677, "Array of States to Process"=w676) -> ("Modified Array of States to Process"=w675:T1)  [unwired: 13 in]
        n332 = local write "state control"(w675) -> ()
        n333 = Increment(x=w693) -> (x+1=w694:i32)
        n334 = Greater Or Equal?(x=w694, y=8000) -> (x >= y?=w687:bool)
        n335 = Increment(x=w691) -> (x+1=w686:i32)
        n336 = Select(t=0, s=w687, f=w686) -> (s? t:f=w684:i32)
        n337 = Greater Or Equal?(x=w686, y=1500) -> (x >= y?=w680:bool)
        n338 = Select(t=T1 "wait position" ("f"), s=w680, f=T1 "check position") -> (s? t:f=w679:T1)
        n339 = case shown="True" w680 {
          tunnel: [w698 0] -> _
          tunnel: [w695 T1[] ["retract out", "insert out", "wait"]] -> w690
          tunnel: [w696 T1 "retract out" ("state control")] -> _
          tunnel: w686 -> [w698 _]
          tunnel: w677 -> [w697 _]
          tunnel: [w697 "rotate failure"] -> w689
          tunnel: w679 -> [w696 _]
          tunnel: w676 -> [w695 _]
          frame False {
          }
          frame True {
          }
        }
      }
      frame "check position" {
        w706 = i16 14  # Encoder Bits
        (unwired) 2794.0 ("y")
        (unwired) 2730.0 ("y")
        (unwired) 2613.0 ("y")
        (unwired) u32 16838 ("x")
        # "Motor Value"
        # "Requested Sample Position Number"
        # "Off-Set"
        n340 = Search 1D Array(1D array=w704, element=T1 "check position") -> (index of element=w748:i32)  [unwired: 1 in]
        n341 = Increment(x=w748) -> (x+1=w747:i32)
        n342 = Index Array(array=w704, index=w747) -> (element=w749:T1)
        n343 = shared-variable "SCA-cRIO\\shared var lib.lvlib\\Encoder Home Off-Set"() -> (w703:dbl)  [unwired: 1 in, 1 out]
        n344 = local read "encoder position"() -> (w734:u16)
        n345 = local write "state control"(w749) -> ()
        n346 = Decrement(x="New Sample") -> (x-1=w708:dbl)
        n347 = Scale By Power Of 2(n=w706, x=u32 1) -> (x*2^n=w705:u32)
        n348 = Subtract(x=64.0, y=w708) -> (x-y=w714:dbl)
        n349 = Multiply(x=w708, y=256.0) -> (x*y=w720:dbl)
        n350 = Add(x=w734, y="Window radius") -> (x+y=w739:u32)
        n351 = Less?(x=w734, y="Window radius") -> (x < y?=w732:bool)
        n352 = Subtract(x=w705, y=w734) -> (x-y=w738:u32)
        n353 = Subtract(x=w734, y="Window radius") -> (x-y=w736:u32)
        n354 = Multiply(x=w714, y=256.0) -> (x*y=w713:dbl)
        n355 = Less?(x=w738, y="Window radius") -> (x < y?=w737:bool)
        n356 = Subtract(x=w705, y=w736) -> (x-y=w733:u32)
        n357 = Add(x=w720, y=w703) -> (x+y=w710:dbl)
        n358 = Greater Or Equal?(x=w708, y=54.0) -> (x >= y?=w712:bool)
        n359 = Subtract(x=w703, y=w713) -> (x-y=w711:dbl)
        n360 = Select(t=w738, s=w737, f=w739) -> (s? t:f=w718:u32)
        "Upper Limit" <- w718
        n361 = Select(t=w733, s=w732, f=w736) -> (s? t:f=w719:u32)
        "Lower Limit" <- w719
        n362 = Select(t=w711, s=w712, f=w710) -> (s? t:f=w709:dbl)
        "Destination (encoder)" <- w709
        n363 = shared-variable "SCA-cRIO\\shared var lib.lvlib\\wheel  value"(w709) -> ()  [unwired: 1 in, 1 out]
        n364 = shared-variable "SCA-cRIO\\shared var lib.lvlib\\wheel offset plus"(w718) -> ()  [unwired: 1 in, 1 out]
        n365 = shared-variable "SCA-cRIO\\shared var lib.lvlib\\wheel offset minus"(w719) -> ()  [unwired: 1 in, 1 out]
        n366 = Subtract(x=w709, y=w734) -> (x-y=w727:dbl)
        n367 = In Range and Coerce(upper limit=w718, x=w709, lower limit=w719) -> (In Range?=w724:bool)  [unwired: 1 out]
        "In Range?" <- w724
        n368 = Select(t=w749, s=w724, f=T1 "rotate wheel") -> (s? t:f=w745:T1)
        n369 = Multiply(x=w727, y=3.0519) -> (x*y=→"Move (motor steps)":dbl)
        n370 = case shown="False" FALSE {
          tunnel: [0 0] -> _
          tunnel: [w751 T1[] ["retract out", "insert out", "wait"]] -> w746
          tunnel: [w752 T1 "retract out" ("state control")] -> w744
          tunnel: w743 -> [w753 _]
          tunnel: [w753 "rotate failure"] -> w742
          tunnel: w745 -> [w752 _]
          tunnel: w704 -> [w751 _]
          frame False {
          }
          frame True {
          }
        }
      }
      frame "quick rotate" {
        w782 = 350 ("y")
        w786 = 1000.0 ("acceleration")
        n371 = Search 1D Array(1D array=w771, element=w767) -> (index of element=w776:i32)  [unwired: 1 in]
        n372 = Increment(x=w783) -> (x+1=w784:i32)
        n373 = Decrement(x=55.0) -> (x-1=w779:dbl)
        n374 = Multiply(x=w779, y=78.125) -> ()  [unwired: 1 out]
        n375 = shared-variable "SCA-cRIO\\shared var lib.lvlib\\encoder set"() -> (w759:dbl)  [unwired: 1 in, 1 out]
        "encoder set value" <- w759
        n376 = Increment(x=w776) -> (x+1=w775:i32)
        n377 = Greater Or Equal?(x=w784, y=w782) -> (x >= y?=w763:bool)
        n378 = Increment(x=w772) -> (x+1=w762:i32)
        n379 = Subtract(x=w782, y=5) -> (x-y=w764:i32)
        n380 = Less Or Equal?(x=w783, y=w764) -> (x <= y?=w780:bool)
        n381 = Index Array(array=w771, index=w775) -> (element=w777:T1)
        n382 = Select(t=0, s=w763, f=w762) -> (s? t:f=w760:i32)
        n383 = Greater Or Equal?(x=w762, y=800) -> (x >= y?=w773:bool)
        n384 = local write "state control"(w777) -> ()
        n385 = Select(t=w777, s=w763, f=w767) -> (s? t:f=w769:T1)
        n386 = xnode "Straight-Line Move"("resource"=w788, "execute"=w780, "position"=w759, "velocity"=w786, "acceleration"=w786, "deceleration"=w786, "accel. jerk"=w786, "smoothing"=w786) -> ("resource out"=w787:refnum<k21>, "done"=→"done 2":bool)  [unwired: 2 in, 4 out]
        n387 = case shown="False" w773 {
          tunnel: [w792 0] -> _
          tunnel: [w789 T1[] ["retract out", "insert out", "wait"]] -> w770
          tunnel: [w790 T1 "retract out" ("state control")] -> w768
          tunnel: w762 -> [w792 _]
          tunnel: w767 -> [w791 _]
          tunnel: [w791 "rotate failure"] -> w766
          tunnel: w769 -> [w790 _]
          tunnel: w771 -> [w789 _]
          frame False {
          }
          frame True {
          }
        }
      }
    }
    "state control 2" <- w278
    "action" <- w273
    n388 = shared-variable "SCA-cRIO\\shared var lib.lvlib\\sc control"(w270) -> ()  [unwired: 1 in, 1 out]
    n389 = shared-variable "SCA-cRIO\\shared var lib.lvlib\\count"(w268) -> ()  [unwired: 1 in, 1 out]
    n390 = node-c288() -> ()  [unwired: 1 in, 1 out]
  }
  n391 = while {
    tunnel: [w852] -> _
    shift-right: [w844] -> _
    shift-left: i16 11 ("indextest") -> [w847]
    tunnel: w33 -> [_]
    tunnel: w12 -> [w843]
    shift-right: [w835] -> _
    shift-left: 0.0 -> [w836]
    stop <- FALSE ("stop") stop-if-true
    n392 = shared-variable "SCA-cRIO\\Mod7\\Sample Rod UP sensor"() -> (w827:bool, error out=w849:errorcluster)  [unwired: 1 in]
    "sample rod UP sensor" <- w827
    n393 = Increment(x=w836) -> (x+1=w835:dbl)
    n394 = local read "end sample test"() -> (w838:bool)
    n395 = shared-variable "SCA-cRIO\\shared var lib.lvlib\\indextest"() -> (w845:i16)  [unwired: 1 in, 1 out]
    n396 = shared-variable "SCA-cRIO\\shared var lib.lvlib\\end test"() -> (w839:bool)  [unwired: 1 in, 1 out]
    n397 = shared-variable "SCA-cRIO\\shared var lib.lvlib\\read rod up"(w827) -> ()  [unwired: 1 in, 1 out]
    n398 = shared-variable "SCA-cRIO\\Mod7\\Sample Rod DOWN sensor"(error in=w849) -> (w828:bool, error out=w848:errorcluster)
    "sample rod DOWN sensor" <- w828
    n399 = Or(x=w839, y=w838) -> (x .or. y?=w837:bool)
    n400 = Equal?(x=w845, y=w847) -> (x = y?=w846:bool)
    n401 = shared-variable "SCA-cRIO\\shared var lib.lvlib\\read rod  down"(w828) -> ()  [unwired: 1 in, 1 out]
    n402 = local write "end sample test"(w837) -> ()
    n403 = shared-variable "SCA-cRIO\\Mod7\\Retract Rod OUT sensor"(error in=w848) -> (w829:bool, error out=w857:errorcluster)
    "retract rod OUT sensor" <- w829
    n404 = xnode "Read\n(Data)"("resource"=w843) -> ("position"=w840:dbl)  [unwired: 1 in, 4 out]
    "position" <- w840
    n405 = shared-variable "SCA-cRIO\\shared var lib.lvlib\\read retract out"(w829) -> ()  [unwired: 1 in, 1 out]
    n406 = shared-variable "SCA-cRIO\\Mod7\\Retract Rod IN sensor"(error in=w857) -> (w830:bool, error out=w856:errorcluster)
    "retract rod IN sensor" <- w830
    n407 = shared-variable "SCA-cRIO\\shared var lib.lvlib\\read retract in"(w830) -> ()  [unwired: 1 in, 1 out]
    n408 = shared-variable "SCA-cRIO\\shared var lib.lvlib\\position"(w840) -> ()  [unwired: 1 in, 1 out]
    n409 = Divide(x=w840, y=78.125) -> (x/y=w841:dbl)
    "wheel position readback" <- w841
    n410 = shared-variable "SCA-cRIO\\Mod7\\Insert Rod OUT sensor"(error in=w856) -> (w831:bool, error out=w855:errorcluster)
    "insert rod OUT sensor" <- w831
    n411 = shared-variable "SCA-cRIO\\shared var lib.lvlib\\wheel readback"(w841) -> ()  [unwired: 1 in, 1 out]
    n412 = shared-variable "SCA-cRIO\\shared var lib.lvlib\\read insert out"(w831) -> ()  [unwired: 1 in, 1 out]
    n413 = case shown="False" w846 {
      tunnel: w845 -> [w872 _]
      tunnel: [i16 11 ("indextest") i16 11 ("indextest")] -> w844
      frame False {
        # "Requested Sample Position Number"
        n414 = shared-variable "SCA-cRIO\\shared var lib.lvlib\\indextest"(i16 0 ("indextest")) -> ()  [unwired: 1 in, 1 out]
        n415 = shared-variable "SCA-cRIO\\shared var lib.lvlib\\sample number"() -> (w868:i16)  [unwired: 1 in, 1 out]
        n416 = property on="state control" class="CmbBox (strict)"() -> ("Strings[]"=w873:string[])  [unwired: 2 in, 2 out]
        n417 = Index Array(array=w873, index=w872) -> (element=→"sc control":string)
        n418 = local write "New Sample"(w868) -> ()
        "indextest" <- w872
      }
      frame True {
      }
    }
    n419 = shared-variable "SCA-cRIO\\shared var lib.lvlib\\change sample start end"() -> (→"change sample start end":bool)  [unwired: 1 in, 1 out]
    n420 = shared-variable "SCA-cRIO\\Mod7\\Insert Rod IN sensor"(error in=w855) -> (w832:bool, error out=w854:errorcluster)
    "insert rod IN sensor" <- w832
    n421 = shared-variable "SCA-cRIO\\shared var lib.lvlib\\start sample change"() -> (→"start sample change":bool)  [unwired: 1 in, 1 out]
    n422 = shared-variable "SCA-cRIO\\shared var lib.lvlib\\read insert in"(w832) -> ()  [unwired: 1 in, 1 out]
    n423 = shared-variable "SCA-cRIO\\Mod7\\Wheel GV CLOSED sensor"(error in=w854) -> (w833:bool, error out=w853:errorcluster)
    "SC GV CLOSED sensor" <- w833
    n424 = Wait Until Next ms Multiple(millisecond multiple=u32 1000) -> ()  [unwired: 1 out]
    n425 = shared-variable "SCA-cRIO\\shared var lib.lvlib\\read sc gv closed"(w833) -> ()  [unwired: 1 in, 1 out]
    n426 = shared-variable "SCA-cRIO\\Mod7\\Wheel GV OPEN sensor"(error in=w853) -> (w834:bool, error out=w852:errorcluster)
    "error out" <- w852
    "SC GV OPEN sensor" <- w834
    n427 = shared-variable "SCA-cRIO\\shared var lib.lvlib\\read sc gv open"(w834) -> ()  [unwired: 1 in, 1 out]
  }
  n428 = while {
    stop <- FALSE stop-if-true
    n429 = shared-variable "SCA-cRIO\\shared var lib.lvlib\\rod up shared"() -> (w876:bool)  [unwired: 1 in, 1 out]
    "set rod up" <- w876
    n430 = Wait Until Next ms Multiple(millisecond multiple=u32 100) -> ()  [unwired: 1 out]
    n431 = case shown="True" w876 {
      frame False {
      }
      frame True {
        n432 = shared-variable "SCA-cRIO\\shared var lib.lvlib\\rod up shared"(FALSE ("rod up shared")) -> ()  [unwired: 1 in, 1 out]
        n433 = local write "state control"(T1 "rod up" ("state control")) -> ()
      }
    }
  }
  n434 = while {
    stop <- FALSE stop-if-true
    n435 = shared-variable "SCA-cRIO\\shared var lib.lvlib\\rotate wheel"() -> (w881:bool)  [unwired: 1 in, 1 out]
    "rotate wheel" <- w881
    n436 = Wait Until Next ms Multiple(millisecond multiple=u32 100) -> ()  [unwired: 1 out]
    n437 = case shown="True" w881 {
      frame False {
      }
      frame True {
        n438 = shared-variable "SCA-cRIO\\shared var lib.lvlib\\rotate wheel"(FALSE ("rod up shared")) -> ()  [unwired: 1 in, 1 out]
        n439 = local write "state control"(T1 "rotate wheel" ("state control")) -> ()
      }
    }
  }
  n440 = while {
    stop <- FALSE stop-if-true
    n441 = shared-variable "SCA-cRIO\\shared var lib.lvlib\\change sample"() -> (w886:bool)  [unwired: 1 in, 1 out]
    "set cold cathode on 2" <- w886
    n442 = Wait Until Next ms Multiple(millisecond multiple=u32 50) -> ()  [unwired: 1 out]
    n443 = case shown="True" w886 {
      frame False {
      }
      frame True {
        n444 = shared-variable "SCA-cRIO\\shared var lib.lvlib\\change sample"(FALSE ("rod up shared")) -> ()  [unwired: 1 in, 1 out]
        n445 = local write "state control"(T1 "change sample" ("state control")) -> ()
      }
    }
  }
  n446 = while {
    stop <- FALSE stop-if-true
    n447 = shared-variable "SCA-cRIO\\shared var lib.lvlib\\set encoder wheel"() -> (w890:bool)  [unwired: 1 in, 1 out]
    n448 = Wait Until Next ms Multiple(millisecond multiple=u32 100) -> ()  [unwired: 1 out]
    n449 = case shown="True" w890 {
      frame False {
      }
      frame True {
        n450 = shared-variable "SCA-cRIO\\shared var lib.lvlib\\set encoder wheel"(FALSE ("rod up shared")) -> ()  [unwired: 1 in, 1 out]
        n451 = local write "state control"(T1 "quick rotate" ("state control")) -> ()
      }
    }
  }
  n452 = while {
    stop <- FALSE stop-if-true
    n453 = shared-variable "SCA-cRIO\\shared var lib.lvlib\\rezero"() -> (w895:bool)  [unwired: 1 in, 1 out]
    n454 = Wait Until Next ms Multiple(millisecond multiple=u32 100) -> ()  [unwired: 1 out]
    n455 = case shown="True" w895 {
      frame False {
      }
      frame True {
        n456 = shared-variable "SCA-cRIO\\shared var lib.lvlib\\rezero"(FALSE ("rod up shared")) -> ()  [unwired: 1 in, 1 out]
        n457 = local write "state control"(T1 "rezero" ("state control")) -> ()
      }
    }
  }
  n458 = while {
    stop <- FALSE stop-if-true
    (unwired) FALSE ("execute")
    n459 = shared-variable "SCA-cRIO\\shared var lib.lvlib\\cathode set"() -> (w904:dbl)  [unwired: 1 in, 1 out]
    "cathode set" <- w904
    n460 = shared-variable "SCA-cRIO\\shared var lib.lvlib\\extractor set"() -> (w908:dbl)  [unwired: 1 in, 1 out]
    "extractor set" <- w908
    n461 = shared-variable "SCA-cRIO\\shared var lib.lvlib\\immersion lens v set"() -> (w900:dbl)  [unwired: 1 in, 1 out]
    n462 = local read "cathode change"() -> (w906:bool)
    n463 = shared-variable "SCA-cRIO\\Mod7\\Sample Rod DOWN sensor"() -> (w907:bool)  [unwired: 1 in, 1 out]
    n464 = shared-variable "SCA-cRIO\\Mod4\\Extractor V set"(w908) -> ()  [unwired: 1 in, 1 out]
    n465 = shared-variable "SCA-cRIO\\Mod4\\Immersion Lens I set"(7.5 ("immersion lens current set")) -> ()  [unwired: 1 in, 1 out]
    n466 = And(x=w907, y=w906) -> (x .and. y?=w905:bool)
    n467 = shared-variable "SCA-cRIO\\Mod4\\Immersion Lens V set"(w900) -> ()  [unwired: 1 in, 1 out]
    n468 = Select(t=w904, s=w905, f=0.0) -> (s? t:f=w902:dbl)
    n469 = shared-variable "SCA-cRIO\\Mod4\\Cathode V set"(w902) -> ()  [unwired: 1 in, 1 out]
    n470 = Wait Until Next ms Multiple(millisecond multiple=u32 100) -> ()  [unwired: 1 out]
  }
  n471 = while {
    stop <- FALSE stop-if-true
    n472 = shared-variable "SCA-cRIO\\shared var lib.lvlib\\set insert out"() -> (w912:bool)  [unwired: 1 in, 1 out]
    "set insert out" <- w912
    n473 = Wait Until Next ms Multiple(millisecond multiple=u32 100) -> ()  [unwired: 1 out]
    n474 = case shown="True" w912 {
      frame False {
      }
      frame True {
        n475 = shared-variable "SCA-cRIO\\shared var lib.lvlib\\set insert out"(FALSE ("rod up shared")) -> ()  [unwired: 1 in, 1 out]
        n476 = local write "state control"(T1 "insert out" ("state control")) -> ()
      }
    }
  }
  n477 = while {
    stop <- FALSE stop-if-true
    n478 = shared-variable "SCA-cRIO\\shared var lib.lvlib\\set rod down"() -> (w917:bool)  [unwired: 1 in, 1 out]
    "set rod down" <- w917
    n479 = Wait Until Next ms Multiple(millisecond multiple=u32 100) -> ()  [unwired: 1 out]
    n480 = case shown="True" w917 {
      frame False {
      }
      frame True {
        n481 = shared-variable "SCA-cRIO\\shared var lib.lvlib\\set rod down"(FALSE ("rod up shared")) -> ()  [unwired: 1 in, 1 out]
        n482 = local write "state control"(T1 "rod down" ("state control")) -> ()
      }
    }
  }
  n483 = while {
    stop <- FALSE stop-if-true
    n484 = shared-variable "SCA-cRIO\\shared var lib.lvlib\\set pump out system"() -> (w922:bool)  [unwired: 1 in, 1 out]
    "set pump out system" <- w922
    n485 = Wait Until Next ms Multiple(millisecond multiple=u32 100) -> ()  [unwired: 1 out]
    n486 = case shown="True" w922 {
      frame False {
      }
      frame True {
        n487 = shared-variable "SCA-cRIO\\shared var lib.lvlib\\set pump out system"(FALSE ("rod up shared")) -> ()  [unwired: 1 in, 1 out]
        n488 = local write "state control"(T1 "pump out source" ("state control")) -> ()
      }
    }
  }
  n489 = while {
    stop <- FALSE stop-if-true
    n490 = shared-variable "SCA-cRIO\\shared var lib.lvlib\\set cold cathode off"() -> (w927:bool)  [unwired: 1 in, 1 out]
    "set cold cathode off" <- w927
    n491 = Wait Until Next ms Multiple(millisecond multiple=u32 100) -> ()  [unwired: 1 out]
    n492 = case shown="True" w927 {
      frame False {
      }
      frame True {
        n493 = shared-variable "SCA-cRIO\\shared var lib.lvlib\\set cold cathode off"(FALSE ("rod up shared")) -> ()  [unwired: 1 in, 1 out]
        n494 = local write "state control"(T1 "turn cold cathode off" ("state control")) -> ()
      }
    }
  }
  n495 = while {
    stop <- FALSE stop-if-true
    n496 = shared-variable "SCA-cRIO\\shared var lib.lvlib\\set sc close"() -> (w932:bool)  [unwired: 1 in, 1 out]
    "set sc close" <- w932
    n497 = Wait Until Next ms Multiple(millisecond multiple=u32 50) -> ()  [unwired: 1 out]
    n498 = case shown="True" w932 {
      frame False {
      }
      frame True {
        n499 = shared-variable "SCA-cRIO\\shared var lib.lvlib\\set sc close"(FALSE ("rod up shared")) -> ()  [unwired: 1 in, 1 out]
        n500 = local write "state control"(T1 "sc gate valve close" ("state control")) -> ()
      }
    }
  }
  n501 = while {
    stop <- FALSE stop-if-true
    n502 = shared-variable "SCA-cRIO\\shared var lib.lvlib\\set retract out"() -> (w937:bool)  [unwired: 1 in, 1 out]
    "set push out rod out" <- w937
    n503 = Wait Until Next ms Multiple(millisecond multiple=u32 100) -> ()  [unwired: 1 out]
    n504 = case shown="True" w937 {
      frame False {
      }
      frame True {
        n505 = shared-variable "SCA-cRIO\\shared var lib.lvlib\\set retract out"(FALSE ("rod up shared")) -> ()  [unwired: 1 in, 1 out]
        n506 = local write "state control"(T1 "retract out" ("state control")) -> ()
      }
    }
  }
  n507 = node-c288(w5) -> ()  [unwired: 1 out]
  n508 = VISA Close(VISA resource name=w21, error in (no error)=w22) -> (error out=→"error out 5":errorcluster)
  n509 = node-c288(w38) -> ()  [unwired: 1 out]
